vi "From 2D Int Tree Data.vi"(11 "Tree Data":refnum<class "Tree Data.lvclass">) -> (2 "2D Int":i64[][](array[numeric]))   [LabVIEW 2017, in "Tree API.lvlib" / "2D Int.lvclass"]
doc: "Extract a 2D Int value from Tree Data type."
uses:
  2D Int.lvclass
  Tree Data/Tree Data.lvclass
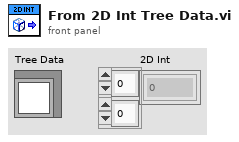
[diagram p1: front panel]
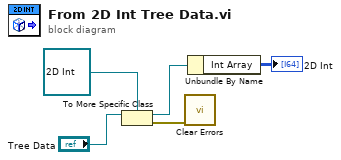
[diagram p0: block diagram]
diagram:
  n1 = To More Specific Class(target class=refnum<class "2D Int.lvclass"> refnum ("Tree API.lvlib:2D Int.lvclass"), reference="Tree Data") -> (specific class reference=w4:refnum<class "2D Int.lvclass">, error out=w3:errorcluster)  [unwired: 1 in]
  n2 = call <vilib>:"Clear Errors.vi"("error in (no error)"=w3) -> ()  [unwired: 5 in, 2 out]
  n3 = Unbundle By Name(w4) -> ("Int Array"=→"2D Int":i64[][])
